vi "Output Data.vi"() -> ()   [LabVIEW 2013]
uses:
  qwtblvlib/TD Quantity.ctl
  <vilib>/Math Plots/2D Math Plots/2D Error Bar/2D Error Bar XCtrl/2D Error Bar.xctl
  <vilib>/Math Plots/3D Math Plots/3D Surface/3D Surface XCtrl/3D Surface.xctl
  globals.vi
  <vilib>/gmath/interp.llb/Create Mesh Grid (2D) (x,y arrays).vi
  <vilib>/Math Plots/3D Math Plots/3D Surface/3D Surface Datatype/Public/Plot Helper (Matrix).vi
  <vilib>/Math Plots/2D Math Plots/2D Error Bar/2D Error Bar Datatype/Public/Plot Helper (Fixed).vi
  <vilib>/Analysis/NI_AALBase.lvlib
  <vilib>/Math Plots/2D Math Plots/2D Error Bar/2D Error Bar Datatype/2D Error Bar Datatype.lvclass
  <vilib>/Math Plots/3D Math Plots/3D Surface/3D Surface Datatype/3D Surface Datatype.lvclass
  <vilib>/gmath/NI_Gmath.lvlib
  qwtblvlib/QWTBLVLib.lvlib
panel:
  in  "redraw quantity signal":bool
  in  "Qtab":enum32{"Raw values", "Graph", "Histogram"}(tab)
  out "Selected Quantity":T1={"Name"="", "Value"=[[1.0]], "Uncertainty"=[[1.0]], "Degrees of\nFreedom"=[[10.0]], "Correlation"=[[10.0]], "Randomized uncertainty"=[[10.0]]}
  out "value 3D":refnum<class "3D Plot Datatype.lvclass">[](xcontrol)
  out "value 2D":refnum<class "2D Plot Datatype.lvclass">[](xcontrol)
  out "value string":string
  out "Histogram Graph":T2(graph)
  out "hist-notOK":string
  in  "new data signal":bool
  in  "Q list":i32(listbox) caption="Input Quantities"
  # "Output data"
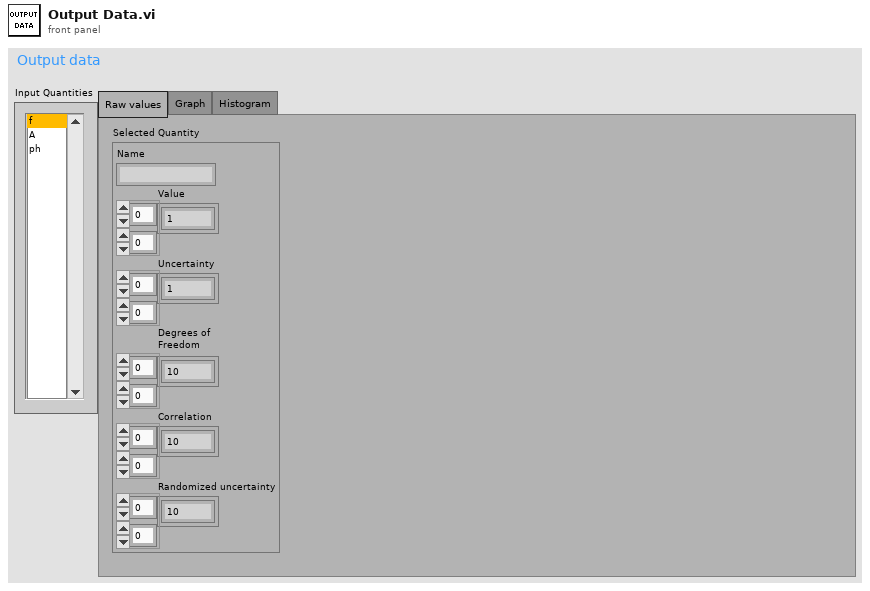
[diagram p1: front panel]
types:
  T1 = typedef "QWTBLVLib.lvlib/TD Quantity.ctl" = cluster{"Name":string, "Value":dbl[][], "Uncertainty":dbl[][], "Degrees of\nFreedom":dbl[][], "Correlation":dbl[][], "Randomized uncertainty":dbl[][]}
  T2 = cluster{"X Values":dbl[], "Histogram: h(x)":i32[]}
  T3 = enum32{"Invalid", "Standard", "Closed", "Hidden", "Minimized", "Maximized"}
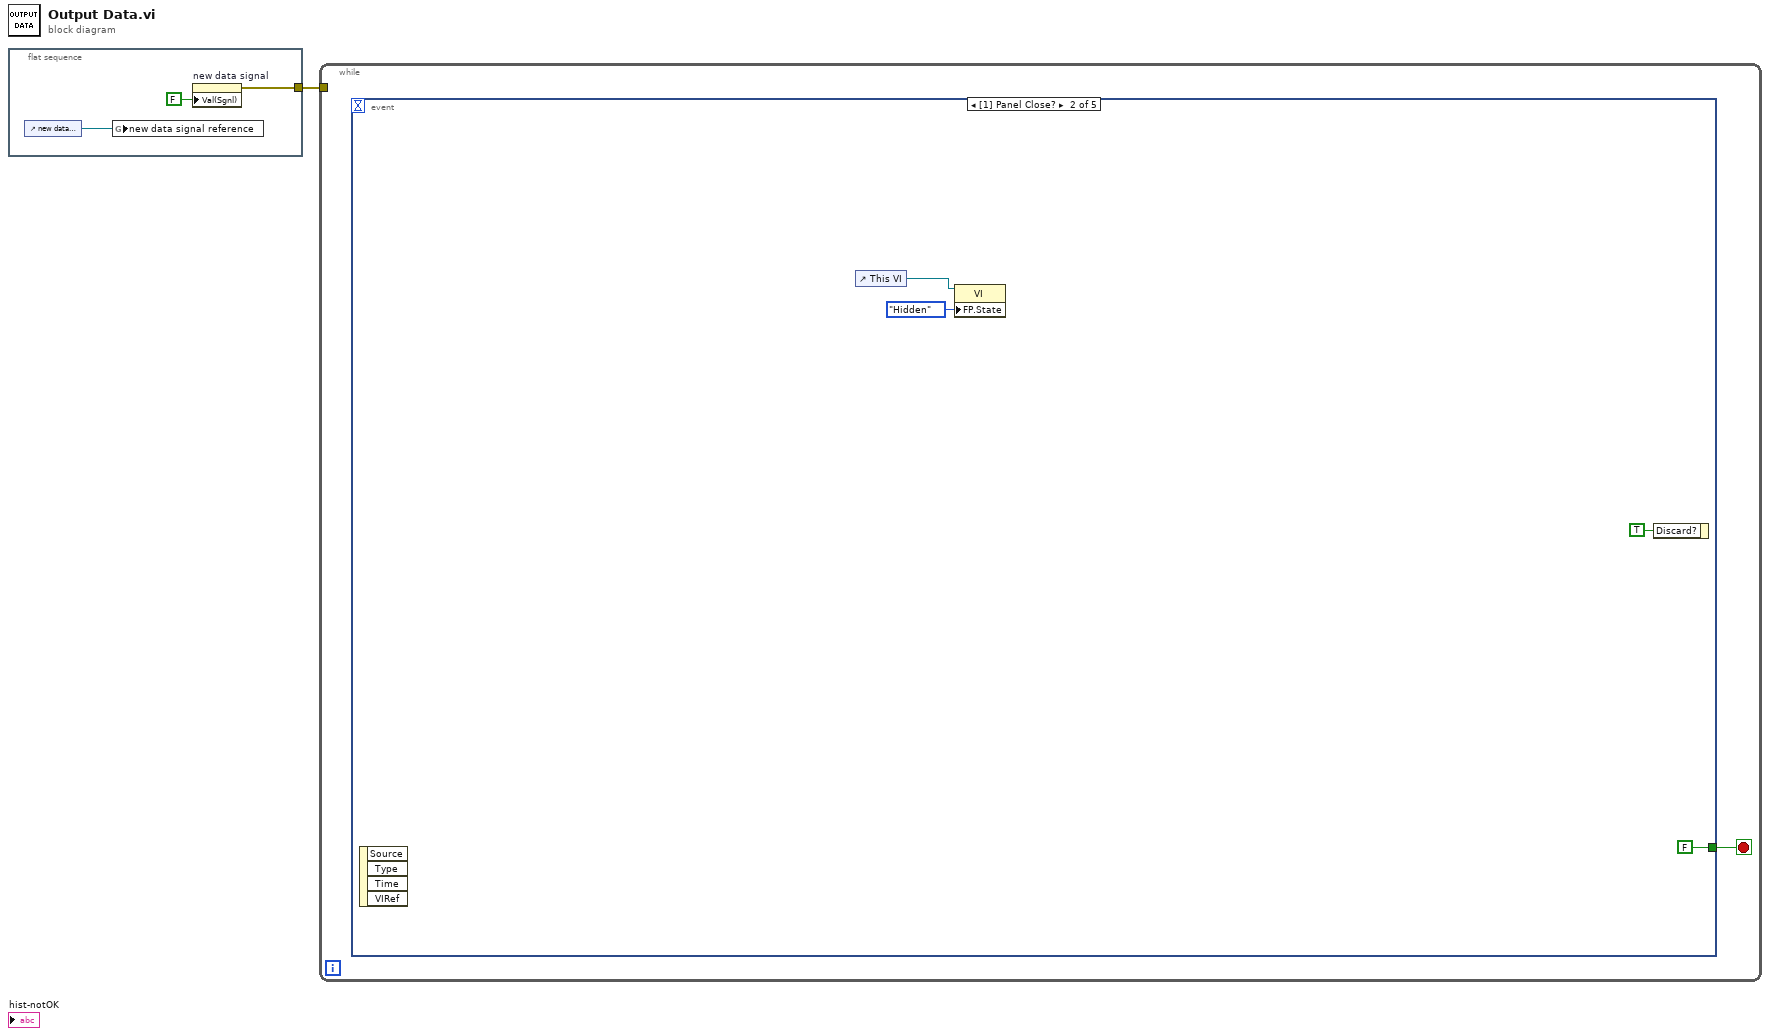
[diagram p0: block diagram]
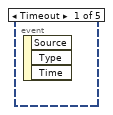
[diagram p2: hidden frame]
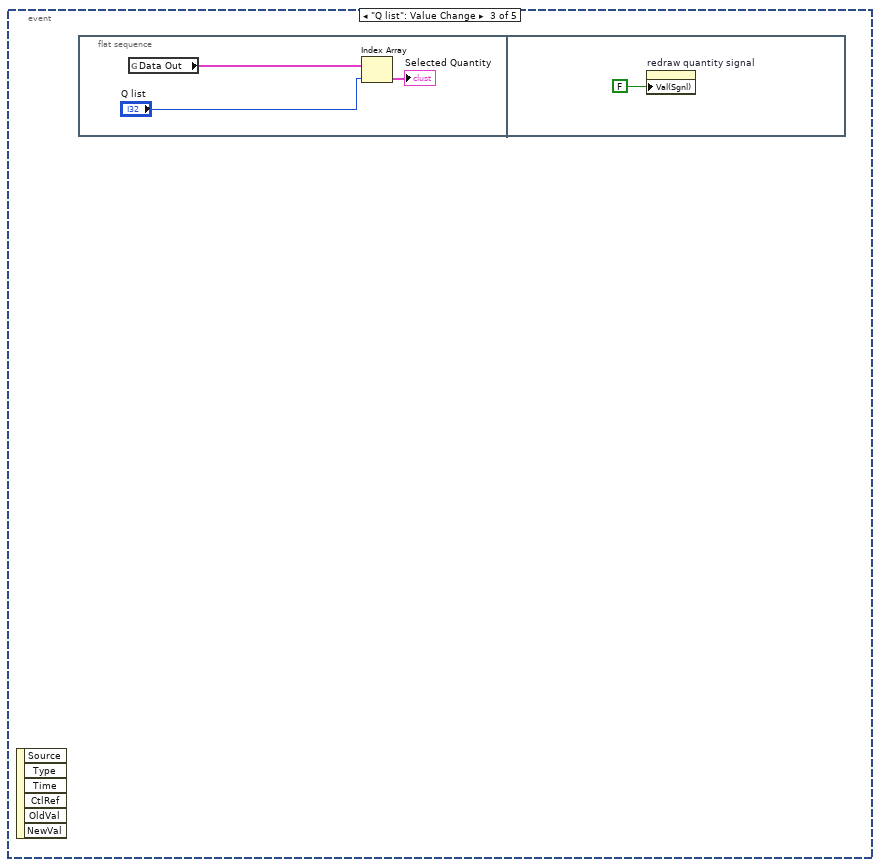
[diagram p3: hidden frame]
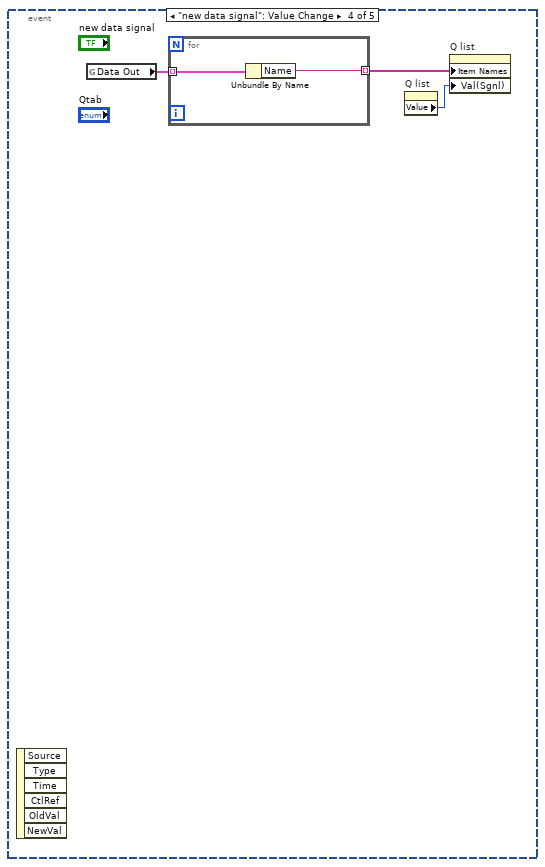
[diagram p4: hidden frame]
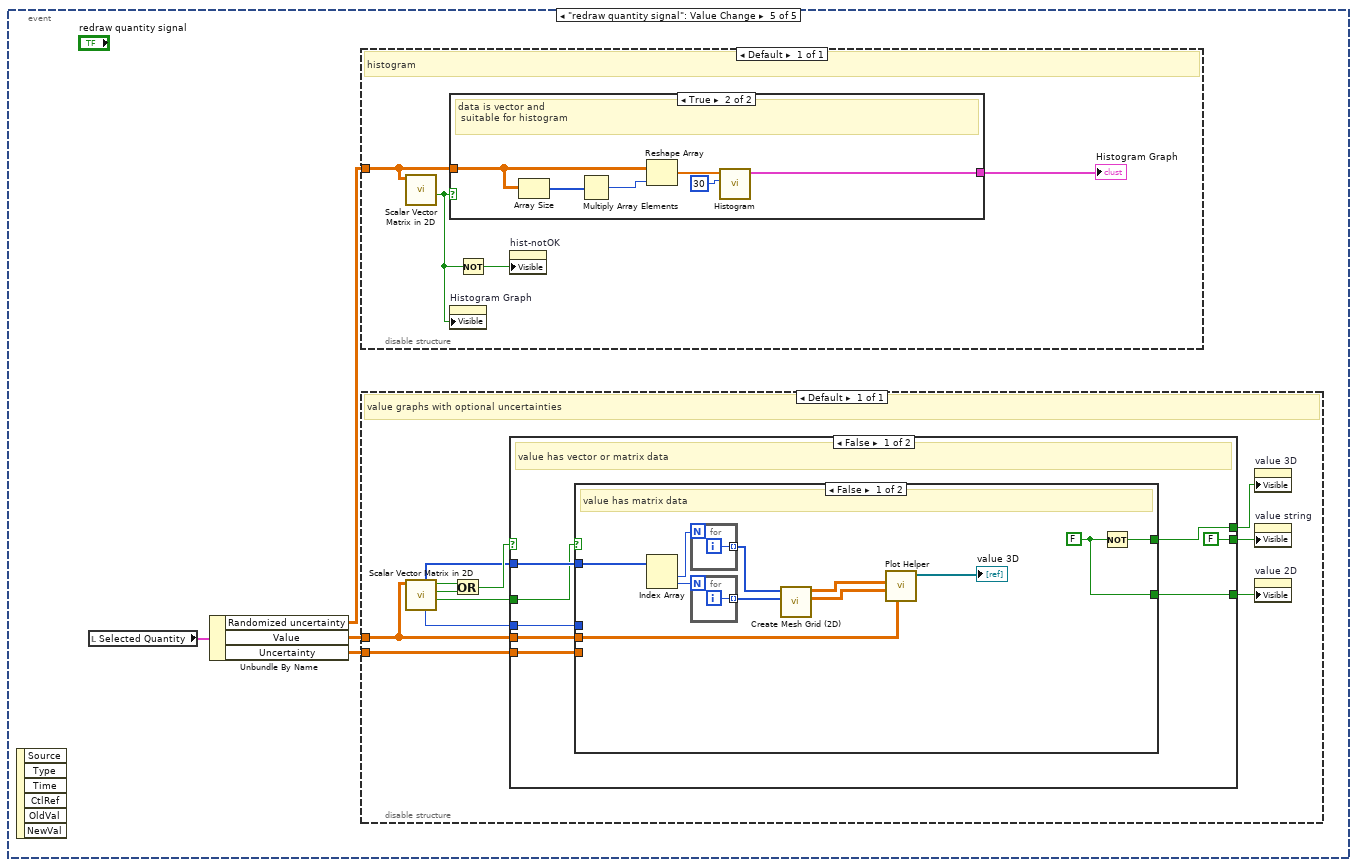
[diagram p5: hidden frame]
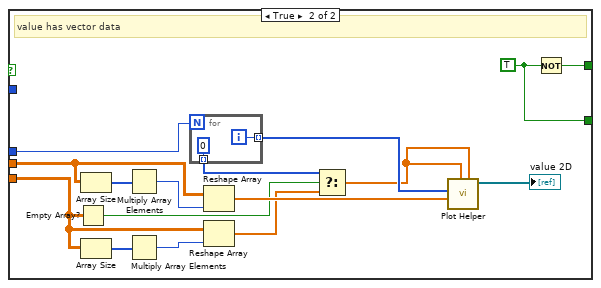
[diagram p6: hidden frame]
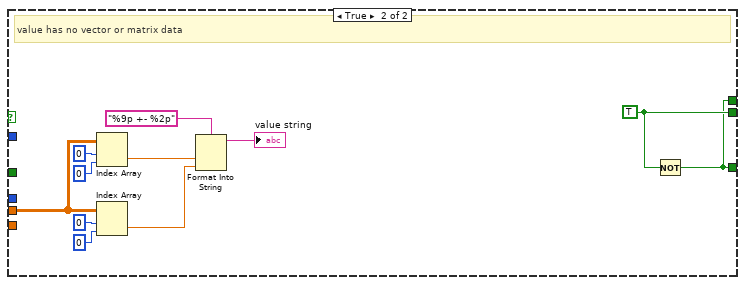
[diagram p7: hidden frame]
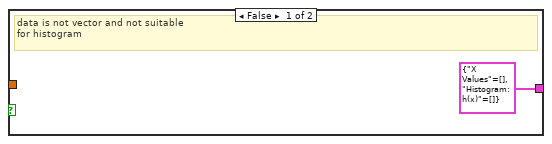
[diagram p8: hidden frame]
diagram:
  n1 = flat-sequence {
    tunnel: [w2] -> w1
    frame #0 {
      n2 = control-ref of="new data signal"() -> (w4:refnum<vi>)
      n3 = global write "globals.vi" "new data signal reference"(w4) -> ()
      n4 = property on="new data signal" class="Bool (strict)"("Val(Sgnl)"=FALSE ("Value (Signaling)")) -> (error out=w2:errorcluster)  [unwired: 2 in, 1 out]
    }
  }
  n5 = while {
    tunnel: w1 -> [_]
    stop <- w5 stop-if-true
    n6 = event shown="[1] Panel Close?" {
      selector: _ -> [_ _ _ _ _]
      dyn-events: _ -> [_ _ _ _ _]
      timeout: _ -> [_ _ _ _ _]
      tunnel: [_ FALSE _ _ _] -> w5
      event Timeout {
        n7 = event-data() -> ()  [unwired: 1 in, 3 out]
      }
      event Panel Close? {
        n8 = event-data() -> ()  [unwired: 1 in, 4 out]
        n9 = control-ref of="This VI"() -> (w7:refnum<vi>)
        n10 = property class="VI"(reference=w7, "FP.State"=T3."Hidden" ("Front Panel Window:State")) -> ()  [unwired: 1 in, 2 out]
        n11 = event-data("Discard?"=TRUE) -> ()  [unwired: 1 in, 1 out]
      }
      event "Q list": Value Change {
        n12 = event-data() -> ()  [unwired: 1 in, 6 out]
        n13 = flat-sequence {
          frame #0 {
            n14 = global read "globals.vi" "Data Out"() -> (w12:T1[])
            n15 = Index Array(array=w12, index="Q list") -> (element=→"Selected Quantity":T1)
          }
          frame #1 {
            n16 = property on="redraw quantity signal" class="Bool (strict)"("Val(Sgnl)"=FALSE ("Value (Signaling)")) -> ()  [unwired: 2 in, 2 out]
          }
        }
      }
      event "new data signal": Value Change {
        n17 = event-data() -> ()  [unwired: 1 in, 6 out]
        n18 = global read "globals.vi" "Data Out"() -> (w16:T1[])
        n19 = for {
          tunnel: [w18] -> w15 mode=indexing
          tunnel: w16 -> [w17] mode=indexing
          n20 = Unbundle By Name(w17) -> ("Name"=w18:string)
        }
        n21 = property on="Q list" class="LstBox (strict)"() -> ("Value"=w14:i32)  [unwired: 2 in, 2 out]
        n22 = property on="Q list" class="LstBox (strict)"("Item Names"=w15, "Val(Sgnl)"=w14) -> ()  [unwired: 2 in, 2 out]
      }
      event "redraw quantity signal": Value Change {
        n23 = event-data() -> ()  [unwired: 1 in, 6 out]
        n24 = local read "Selected Quantity"() -> (w22:T1)
        n25 = Unbundle By Name(w22) -> ("Randomized uncertainty"=w21:dbl[][], "Value"=w20:dbl[][], "Uncertainty"=w19:dbl[][])
        n26 = disable-structure shown="Default" {
          disable-tunnel: w21 -> [w85]
          frame Enabled {
            # "histogram"
            n27 = call "Scalar Vector Matrix in 2D.vi"("2D Array"=w85) -> ("Is Vector?"=w84:bool)  [unwired: 4 in, 6 out]
            n28 = case shown="True" w84 {
              tunnel: [T2 {"X Values"=[], "Histogram: h(x)"=[]} ("Histogram Graph") w94] -> w86
              tunnel: w85 -> [_ w90]
              frame False {
                # "data is not vector and not suitable\nfor histogram"
              }
              frame True {
                # "data is vector and\n suitable for histogram"
                n29 = Array Size(array=w90) -> (size(s)=w91:i32[])
                n30 = Multiply Array Elements(1:w91) -> (0:w89:i32)
                n31 = Reshape Array(w90, w89) -> (w92:dbl[])
                n32 = call <vilib>:"Histogram.vi"("intervals"=30, "X"=w92) -> ("Histogram Graph"=w94:T2)  [unwired: 6 in, 3 out]
              }
            }
            "Histogram Graph" <- w86
            n33 = property on="Histogram Graph" class="XYGraph (strict)"("Visible"=w84) -> ()  [unwired: 2 in, 2 out]
            n34 = Not(x=w84) -> (.not. x?=w87:bool)
            n35 = property on="hist-notOK" class="Str"("Visible"=w87) -> ()  [unwired: 2 in, 2 out]
          }
        }
        n36 = disable-structure shown="Default" {
          disable-tunnel: w20 -> [w30]
          disable-tunnel: w19 -> [w29]
          frame Enabled {
            # "value graphs with optional uncertainties"
            n37 = call "Scalar Vector Matrix in 2D.vi"("2D Array"=w30) -> ("Is Vector?"=w25:bool, "Is Scalar?"=w27:bool, "Is Empty?"=w28:bool, "Dim Max"=w24:i32, "Dimensions"=w23:i32[])  [unwired: 4 in, 2 out]
            n38 = Or(x=w28, y=w27) -> (x .or. y?=w26:bool)
            n39 = case shown="False" w26 {
              tunnel: [FALSE ("Visible") w83] -> w33
              tunnel: [w39 w82] -> w32
              tunnel: [w40 w82] -> w31
              tunnel: w30 -> [w38 w75]
              tunnel: w23 -> [w37 _]
              tunnel: w29 -> [w36 _]
              tunnel: w25 -> [w35 _]
              tunnel: w24 -> [w34 _]
              frame False {
                # "value has vector or matrix data"
                n40 = case shown="False" w35 {
                  tunnel: [w51 w60] -> w40
                  tunnel: [w52 w61] -> w39
                  tunnel: w38 -> [w49 w66]
                  tunnel: w37 -> [w46 _]
                  tunnel: w34 -> [_ w68]
                  tunnel: w36 -> [_ w59]
                  frame False {
                    w51 = FALSE ("Visible")
                    # "value has matrix data"
                    n41 = Index Array(array=w46) -> (element #1=w42:i32, element #2=w45:i32)  [unwired: 2 in]
                    n42 = for {
                      N: w42 -> [_]
                      tunnel: [w53] -> w43 mode=indexing
                      i -> [w53]
                    }
                    n43 = for {
                      N: w45 -> [_]
                      tunnel: [w54] -> w44 mode=indexing
                      i -> [w54]
                    }
                    n44 = call-poly <vilib>:"Create Mesh Grid (2D).vi"("y domain"=w44, "x domain"=w43) -> ("Y"=w47:dbl[][], "X"=w48:dbl[][])  [unwired: 7 in, 1 out]
                    n45 = call-poly <vilib>:"Plot Helper.vi"("z matrix"=w49, "y matrix"=w47, "x matrix"=w48) -> ("3D Plot lvclass Array out"=→"value 3D":refnum<class "3D Plot Datatype.lvclass">[])  [unwired: 3 in, 5 out]
                    n46 = Not(x=w51) -> (.not. x?=w52:bool)
                  }
                  frame True {
                    w60 = TRUE ("Visible")
                    # "value has vector data"
                    n47 = Empty Array?(array=w59) -> (empty?=w58:bool)
                    n48 = Array Size(array=w66) -> (size(s)=w65:i32[])
                    n49 = Array Size(array=w59) -> (size(s)=w63:i32[])
                    n50 = Multiply Array Elements(1:w65) -> (0:w64:i32)
                    n51 = Multiply Array Elements(1:w63) -> (0:w62:i32)
                    n52 = for {
                      N: w68 -> [_]
                      tunnel: [w72] -> w67 mode=indexing
                      tunnel: [0 ("product")] -> w57 mode=indexing
                      i -> [w72]
                    }
                    n53 = Reshape Array(w66, w64) -> (w69:dbl[])
                    n54 = Reshape Array(w59, w62) -> (w56:dbl[])
                    n55 = Select(t=w57, s=w58, f=w56) -> (s? t:f=w55:dbl[])
                    n56 = call-poly <vilib>:"Plot Helper.vi"("error b vector"=w55, "error a vector"=w55, "y vector"=w69, "x vector"=w67) -> ("2D Plot Class Obj Array out"=→"value 2D":refnum<class "2D Plot Datatype.lvclass">[])  [unwired: 2 in, 5 out]
                    n57 = Not(x=w60) -> (.not. x?=w61:bool)
                  }
                }
              }
              frame True {
                w83 = TRUE ("Visible")
                # "value has no vector or matrix data"
                n58 = Index Array(array=w75, index (row)=0, index (col)=0 ("disabled index (col)")) -> (element=w78:dbl)
                n59 = Index Array(array=w75, index (row)=0, index (col)=0 ("disabled index (col)")) -> (element=w74:dbl)
                n60 = Format Into String(format string="%9p +- %2p", w78, w74) -> (resulting string=→"value string":string)  [unwired: 2 in, 1 out]
                n61 = Not(x=w83) -> (.not. x?=w82:bool)
              }
            }
            n62 = property on="value 3D" class="3D Surface (strict)"("Visible"=w32) -> ()  [unwired: 2 in, 2 out]
            n63 = property on="value string" class="Str"("Visible"=w33) -> ()  [unwired: 2 in, 2 out]
            n64 = property on="value 2D" class="2D Error Bar (strict)"("Visible"=w31) -> ()  [unwired: 2 in, 2 out]
          }
        }
      }
    }
  }
